vi "Main.vi"(8 "error in":errorcluster, 11 "Second Level Worker in":refnum<class "Second Level Worker.lvclass">) -> (0 "error out":errorcluster, 3 "Second Level Worker out":refnum<class "Second Level Worker.lvclass">)   [LabVIEW 2017, in "Method 3.lvlib" / "Second Level Worker.lvclass"]
doc: "The <b>Queued Message Handler</b> of the Worker that owns this VI."
uses:
  Second Level Worker.lvclass
  C:/Program Files (x86)/National Instruments/LabVIEW 2017/vi.lib/addons/_Workers/Library/Classes/Worker/Worker.lvclass
  Initialization Data.ctl
  Response Cases.ctl
  Second Level Worker.lvclass/Second Level Worker.ctl
  rql_Send Error to Caller.ctl
  Base Classes/Worker Base Class/Worker Base Class.lvclass
  <vilib>/addons/_Workers/Library/Classes/Worker/Worker.lvclass
  <vilib>/addons/_Workers/Library/Classes/Message Queue/Message Queue.lvclass
panel:
  in  "Send Error to Caller":bool
  in  "User Error":errorcluster={"status"=TRUE, "code"=12345, "source"="Hello World! This is an error message."}
  # "Method 3 : Using a recursive Public API Request in a base class"
  # "Second Level Worker (Main VI)"
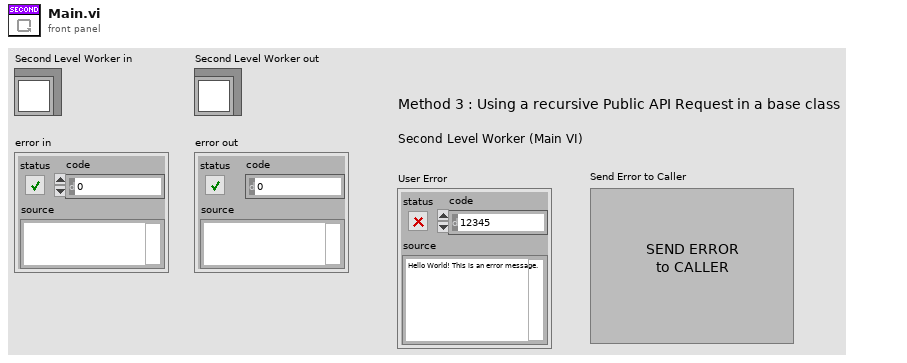
[diagram p1: front panel]
types:
  T1 = typedef "Method 3.lvlib/Second Level Worker.lvclass/Initialization Data.ctl" = cluster{"Response Cases":T2}
  T2 = typedef "Method 3.lvlib/Second Level Worker.lvclass/Response Cases.ctl" = cluster{"Placeholder - Can be deleted":string}
  T3 = typedef "Method 3.lvlib/Second Level Worker.lvclass/rql_Send Error to Caller.ctl" = cluster{"String":string}
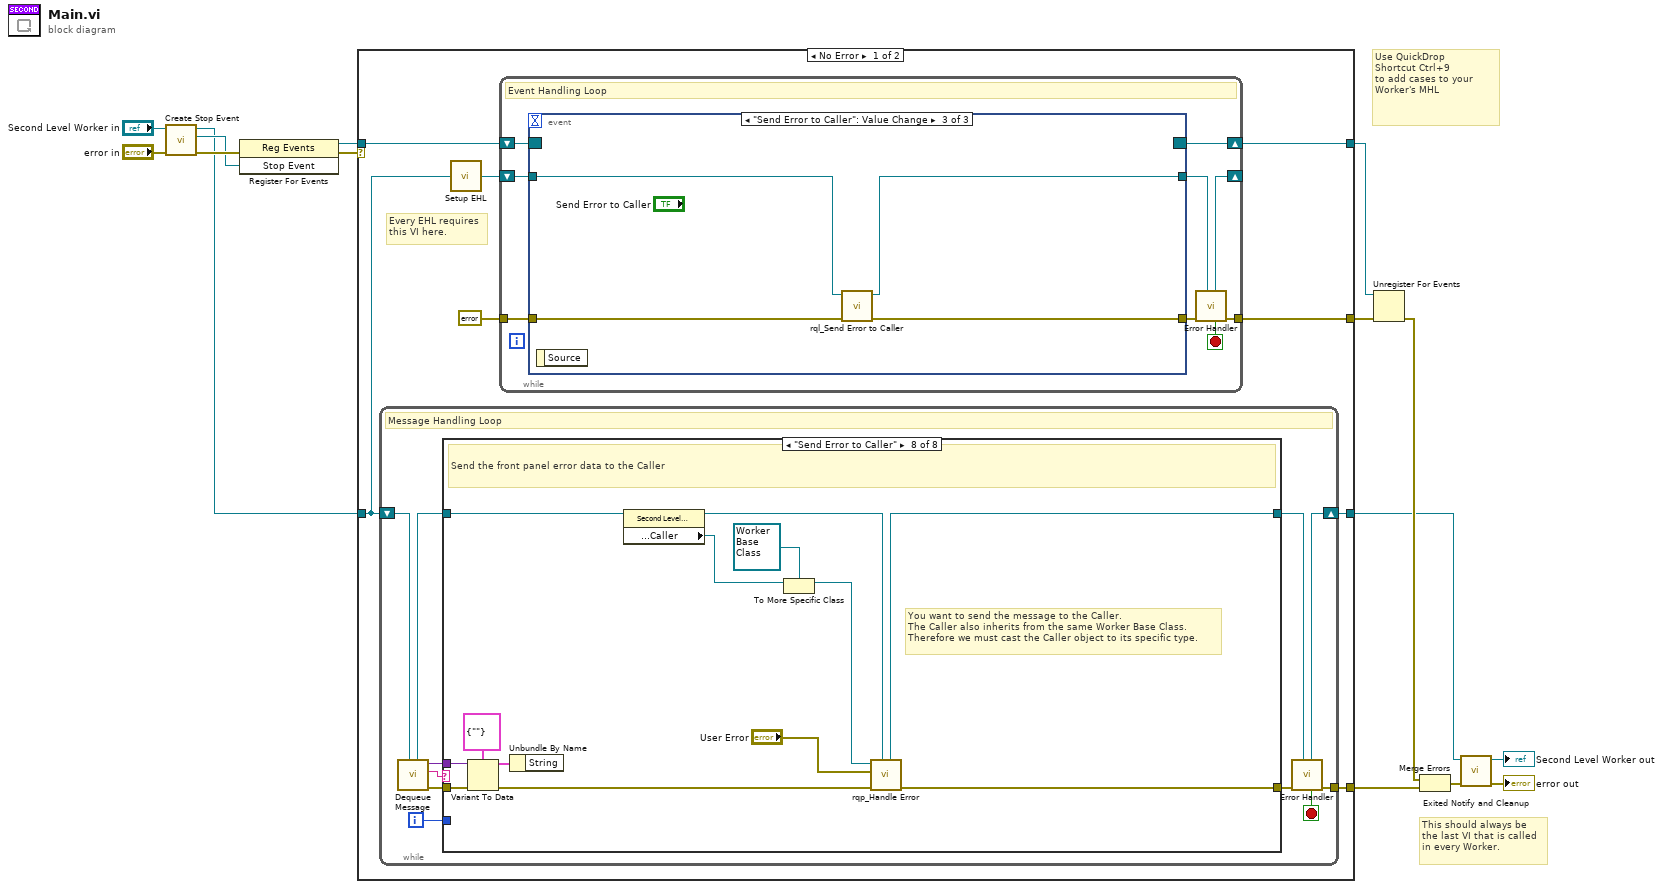
[diagram p0: block diagram]
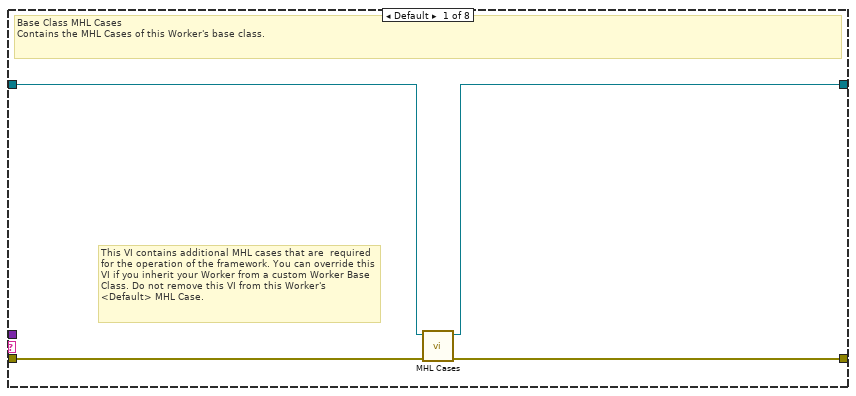
[diagram p2: hidden frame]
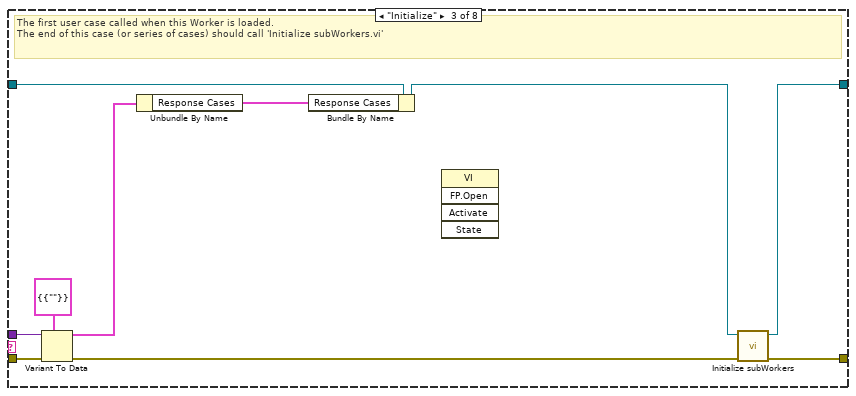
[diagram p4: hidden frame]
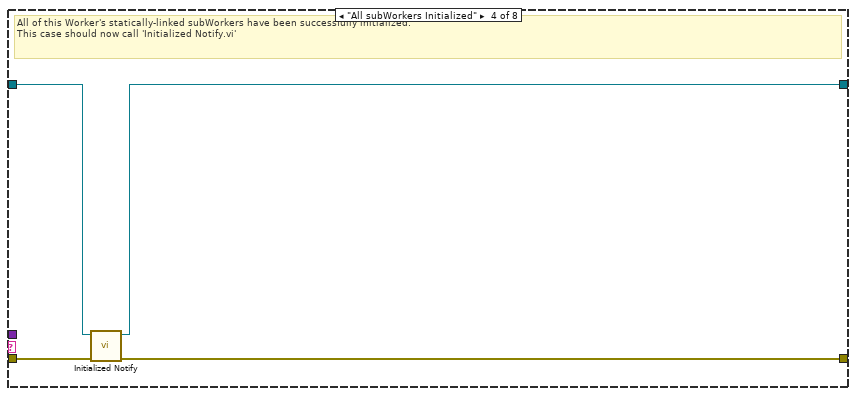
[diagram p5: hidden frame]
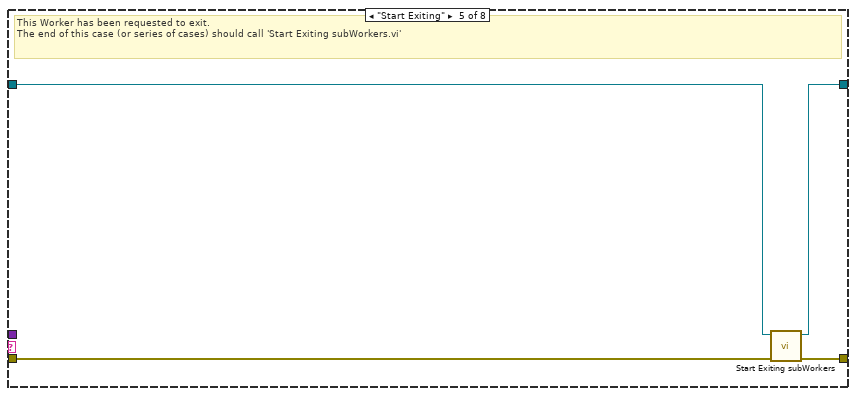
[diagram p6: hidden frame]
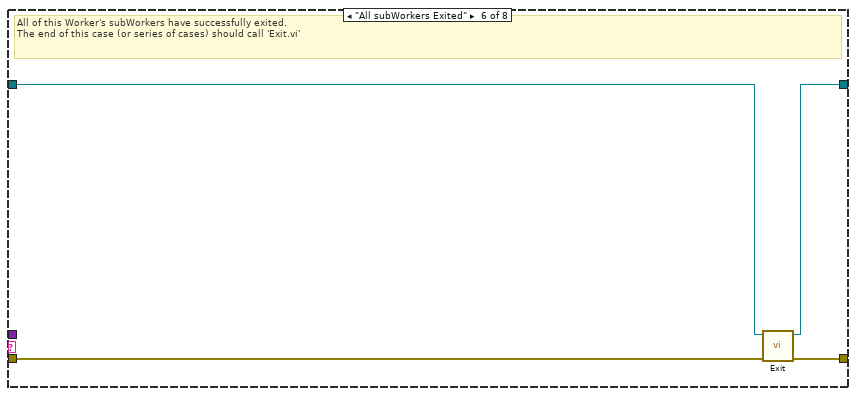
[diagram p7: hidden frame]
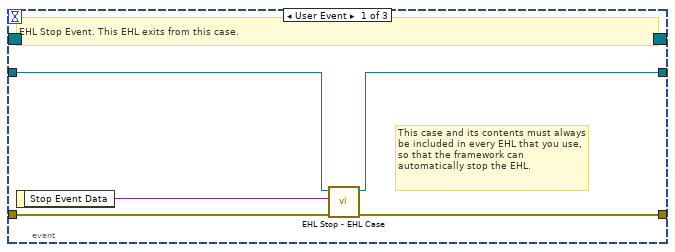
[diagram p9: hidden frame]
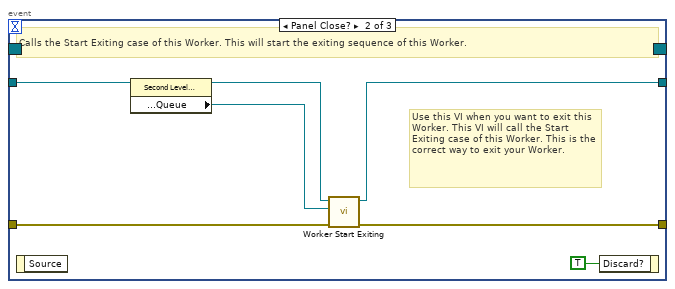
[diagram p10: hidden frame]
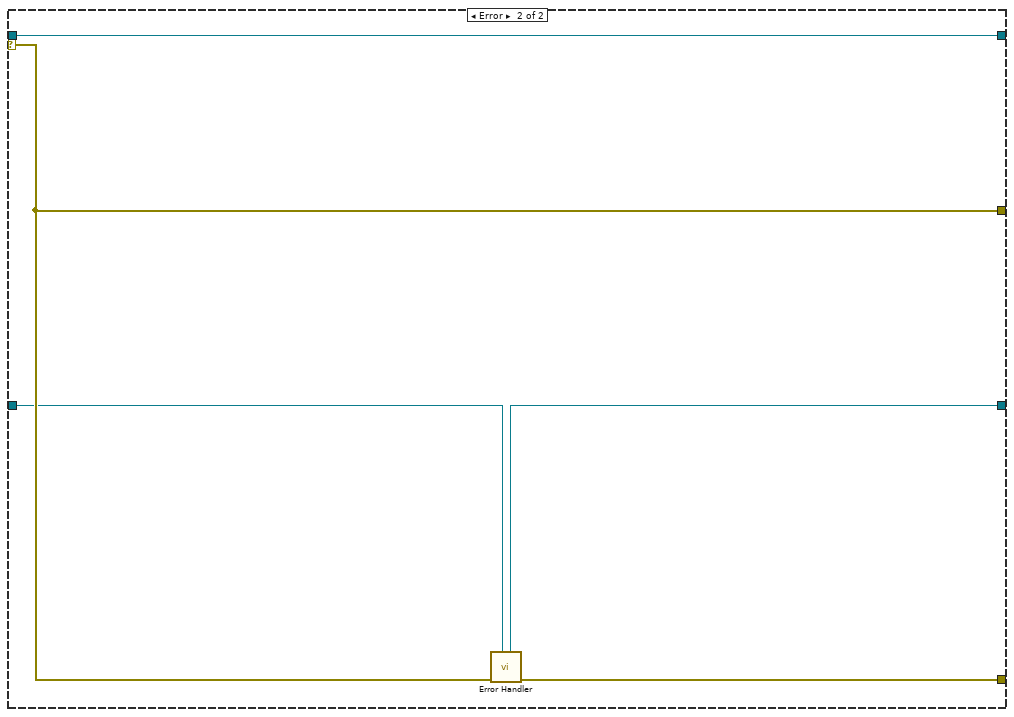
[diagram p11: hidden frame]
diagram:
  # "Use QuickDrop\nShortcut Ctrl+9\nto add cases to your\nWorker's MHL"
  # "This should always be the last VI that is called in every Worker."
  n1 = call-dynamic "Create Stop Event.vi"("error in"="error in", "Worker"="Second Level Worker in") -> ("error out"=w10:errorcluster, "Stop Event"=w7:refnum<user-event>, "Worker out"=w4:refnum<class "Second Level Worker.lvclass">)  [unwired: 7 in]
  n2 = register-events(error in=w10, w7) -> (reference out=w9:refnum<event-registration>, error out=w1:errorcluster)  [unwired: 1 in]
  n3 = case shown="No Error" w1 {
    tunnel: w4 -> [w18 w104]
    tunnel: [w16 w105] -> w8
    tunnel: w9 -> [w23 w106]
    tunnel: [w20 w107] -> w14
    tunnel: [w22 w106] -> w13
    tunnel: [w17 w103] -> w11
    selector: w1 -> [_ w107]
    frame No Error {
      # "Every EHL requires\nthis VI here."
      n4 = while {
        shift-right: [w32] -> w17
        shift-left: w18 -> [w34]
        tunnel: [w33] -> w16
        i -> [w25]
        stop <- w26 stop-if-true
        # "Message Handling Loop"
        n5 = call-dynamic "Dequeue Message.vi"("Worker"=w34) -> ("error out"=w31:errorcluster, "Case out"=w27:string, "Data out"=w24:variant, "Worker out"=w29:refnum<class "Second Level Worker.lvclass">)  [unwired: 6 in, 1 out]
        n6 = case "Worker MHL Case Structure (DO NOT CHANGE LABEL NAME)" shown="\"Send Error to Caller\"" w27 {
          tunnel: w31 -> [w38 w39 w48 w52 w55 w62 w64 w77]
          tunnel: [w37 w39 w50 w51 w58 w61 w64 w73] -> w30
          tunnel: w29 -> [w36 w40 w47 w54 w56 w60 w63 w72]
          tunnel: [w35 w40 w49 w53 w57 w59 w63 w71] -> w28
          tunnel: w25 -> [_ _ _ _ _ _ _ _]
          tunnel: w24 -> [_ _ w45 _ _ _ _ w75]
          frame Default {
            # "This VI contains additional MHL cases that are  required for the operation of the framework. You can override this VI if you inherit your Worker from a custom Worker Base Class. Do not remove this VI from this Worker's <Default> MHL Case."
            # "Base Class MHL Cases\nContains the MHL Cases of this Worker's base class."
            n7 = call-dynamic "MHL Cases.vi"("error in"=w38, "Worker Base Class in"=w36) -> ("error out"=w37:errorcluster, "Worker Base Class out"=w35:refnum<class "Second Level Worker.lvclass">)  [unwired: 8 in]
          }
          frame "------------ FRAMEWORK CASES -----------" {
            # "Start of Workers Framework Cases"
          }
          frame "Initialize" {
            # "The first user case called when this Worker is loaded.\nThe end of this case (or series of cases) should call 'Initialize subWorkers.vi'"
            n8 = Variant To Data(error in=w48, type=T1 {"Response Cases"={"Placeholder - Can be deleted"=""}} ("Initialization Data"), Variant=w45) -> (data=w43:T1, error out=w46:errorcluster)
            n9 = Unbundle By Name(w43) -> ("Response Cases"=w42:T2)
            n10 = Bundle By Name(cluster=w47, "Response Cases"=w42) -> (w44:refnum<class "Second Level Worker.lvclass">)
            n11 = invoke class="VI" method="FP.Open"() -> ()  [unwired: 5 in, 5 out]
            n12 = call-dynamic "Initialize subWorkers.vi"("error in"=w46, "Worker"=w44) -> ("error out"=w50:errorcluster, "dup Worker out"=w49:refnum<class "Second Level Worker.lvclass">)  [unwired: 8 in]
          }
          frame "All subWorkers Initialized" {
            # "All of this Worker's statically-linked subWorkers have been successfully initialized.\nThis case should now call 'Initialized Notify.vi'"
            n13 = call-dynamic "Initialized Notify.vi"("error in"=w52, "Worker"=w54) -> ("error out"=w51:errorcluster, "dup Worker out"=w53:refnum<class "Second Level Worker.lvclass">)  [unwired: 8 in]
          }
          frame "Start Exiting" {
            # "This Worker has been requested to exit. \nThe end of this case (or series of cases) should call 'Start Exiting subWorkers.vi'"
            n14 = call-dynamic "Start Exiting subWorkers.vi"("error_in"=w55, "Worker"=w56) -> ("error out"=w58:errorcluster, "dup Worker out"=w57:refnum<class "Second Level Worker.lvclass">)  [unwired: 8 in]
          }
          frame "All subWorkers Exited" {
            # "All of this Worker's subWorkers have successfully exited. \nThe end of this case (or series of cases) should call 'Exit.vi'"
            n15 = call-dynamic "Exit.vi"("error_in"=w62, "Worker"=w60) -> ("error out"=w61:errorcluster, "dup Worker out"=w59:refnum<class "Second Level Worker.lvclass">)  [unwired: 8 in]
          }
          frame "------------- LOCAL API CASES -------------" {
            # "Start of Workers Local API Cases"
          }
          frame "Send Error to Caller" {
            # "You want to send the message to the Caller.\nThe Caller also inherits from the same Worker Base Class.\nTherefore we must cast the Caller object to its specific type."
            # "Send the front panel error data to the Caller"
            n16 = Variant To Data(error in=w77, type=T3 {"String"=""} ("Data"), Variant=w75) -> (data=w74:T3, error out=w66:errorcluster)
            n17 = Unbundle By Name(w74) -> ()  [unwired: 1 out]
            n18 = property class="Second Level Worker"(reference=w72) -> (reference out=w70:refnum<class "Second Level Worker.lvclass">, "Accessors:Read:Public API:Caller"=w69:refnum<class "Worker.lvclass">)  [unwired: 1 in, 1 out]
            n19 = To More Specific Class(target class=refnum<class "Worker Base Class.lvclass"> refnum ("Worker Base Class"), reference=w69) -> (specific class reference=w67:refnum<class "Worker Base Class.lvclass">)  [unwired: 1 in, 1 out]
            n20 = call "rqp_Handle Error.vi"("Caller in"=w70, "error in"=w66, "Data in"="User Error", "Worker Base Class in"=w67) -> ("error out"=w73:errorcluster, "dup Caller out"=w71:refnum<class "Second Level Worker.lvclass">)  [unwired: 5 in, 1 out]
          }
        }
        n21 = call-dynamic "Error Handler.vi"("Worker"=w28, "error_in"=w30) -> ("error out"=w33:errorcluster, "Stop Loop"=w26:bool, "Worker out"=w32:refnum<class "Second Level Worker.lvclass">)  [unwired: 7 in]
      }
      n22 = call-dynamic "Setup EHL.vi"("Worker"=w18) -> ("Worker out"=w19:refnum<class "Second Level Worker.lvclass">)  [unwired: 14 in]
      n23 = while "Event Handling Loop" {
        shift-right: [w86] -> w22
        shift-left: w23 -> [w85]
        tunnel: [w81] -> w20
        tunnel: errorcluster {"status"=FALSE, "code"=0, "source"=""} ("error constant") -> [w83]
        shift-right: [w79] -> _
        shift-left: w19 -> [w84]
        stop <- w78 stop-if-true
        # "Event Handling Loop"
        n24 = event shown="[2] \"Send Error to Caller\": Value Change" {
          selector: w85 -> [_ _ _]
          dyn-events: [_ _ _] -> w86
          timeout: _ -> [_ _ _]
          tunnel: [w90 w97 w101] -> w82
          tunnel: w83 -> [w91 w96 w102]
          tunnel: w84 -> [w89 w95 w100]
          tunnel: [w88 w94 w99] -> w80
          event User Event {
            # "This case and its contents must always be included in every EHL that you use, so that the framework can automatically stop the EHL."
            # "EHL Stop Event. This EHL exits from this case."
            n25 = event-data() -> ("Stop Event Data"=w87:variant)  [unwired: 1 in]
            n26 = call-dynamic "EHL Stop - EHL Case.vi"("error in"=w91, "Stop Event Data"=w87, "Worker"=w89) -> ("error out"=w90:errorcluster, "Worker out"=w88:refnum<class "Second Level Worker.lvclass">)  [unwired: 7 in]
          }
          event Panel Close? {
            # "Use this VI when you want to exit this Worker. This VI will call the Start Exiting case of this Worker. This is the correct way to exit your Worker."
            # "Calls the Start Exiting case of this Worker. This will start the exiting sequence of this Worker."
            n27 = event-data() -> ()  [unwired: 1 in, 1 out]
            n28 = property class="Second Level Worker"(reference=w95) -> (reference out=w93:refnum<class "Second Level Worker.lvclass">, "Accessors:Read:Public API:Queue"=w92:refnum<class "Message Queue.lvclass">)  [unwired: 1 in, 1 out]
            n29 = call-dynamic "Worker Start Exiting.vi"("error_in"=w96, "Message Queue"=w92, "Worker"=w93) -> ("error out"=w97:errorcluster, "dup Worker out"=w94:refnum<class "Second Level Worker.lvclass">)  [unwired: 7 in]
            n30 = event-data("Discard?"=TRUE) -> ()  [unwired: 1 in, 1 out]
          }
          event "Send Error to Caller": Value Change {
            n31 = event-data() -> ()  [unwired: 1 in, 1 out]
            n32 = call "rql_Send Error to Caller.vi"("error in"=w102, "Second Level Worker in"=w100) -> ("error out"=w101:errorcluster, "dup Second Level Worker out"=w99:refnum<class "Second Level Worker.lvclass">)  [unwired: 8 in]
          }
        }
        n33 = call-dynamic "Error Handler.vi"("Worker"=w80, "error_in"=w82) -> ("error out"=w81:errorcluster, "Stop Loop"=w78:bool, "Worker out"=w79:refnum<class "Second Level Worker.lvclass">)  [unwired: 7 in]
      }
    }
    frame Error {
      n34 = call-dynamic "Error Handler.vi"("Worker"=w104, "error_in"=w107) -> ("error out"=w105:errorcluster, "Worker out"=w103:refnum<class "Second Level Worker.lvclass">)  [unwired: 7 in, 1 out]
    }
  }
  n35 = Unregister For Events(event registration refnum=w13, error in=w14) -> (error out=w15:errorcluster)
  n36 = Merge Errors(w15, w8) -> (w12:errorcluster)
  n37 = call-dynamic "Exited Notify and Cleanup.vi"("error_in"=w12, "Worker"=w11) -> ("error out"=→"error out":errorcluster, "dup Worker out"=→"Second Level Worker out":refnum<class "Second Level Worker.lvclass">)  [unwired: 8 in]
